vi "GT Get Prf Vel.vi"(6 "pClock":u32, 7 "count":i16, 8 "error in (no error)":errorcluster caption="错误输入（无错误）", 10 "profile":i16, 11 "cardNum":i16) -> (0 "error out":errorcluster caption="错误输出", 1 "pValue out":dbl[](array[numeric]), 3 "function return":i16, 4 "pClock out":u32)   [LabVIEW 2014, in "gts.lvlib"]
doc: "GT_API GT_GetPrfVel(short cardNum,short profile,double *pValue,short count=1,unsigned long *pClock=NULL);"
uses:
  gts.lvlib
  gts.dll
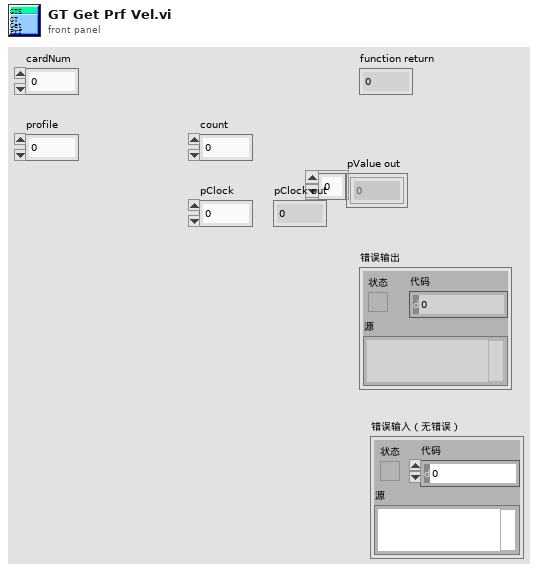
[diagram p1: front panel]
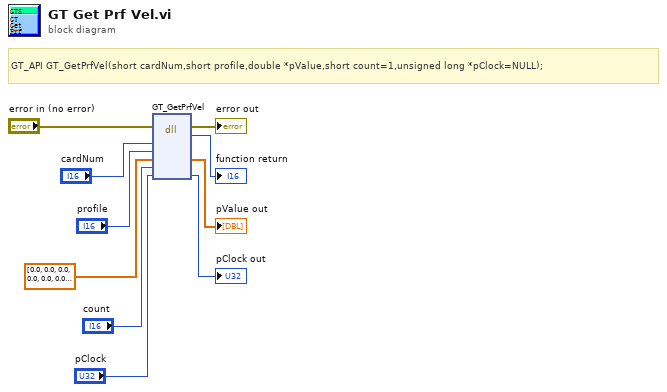
[diagram p0: block diagram]
diagram:
  # "GT_API GT_GetPrfVel(short cardNum,short profile,double *pValue,short count=1,unsigned long *pClock=NULL);"
  n1 = dll-call lib="PTH2?abs D\t王淼清$控制卡常用功能例程(Labview)gts.*" fn="GT_GetPrfVel"(error in="error in (no error)", "cardNum"="cardNum", "profile"="profile", "pValue"=dbl[] [0.0, 0.0, 0.0, 0.0, 0.0, 0.0, 0.0, 1.0], "count"="count", "pClock"="pClock") -> (error out=→"error out":errorcluster, "返回类型"=→"function return":i16, "pValue"=→"pValue out":dbl[], "pClock"=→"pClock out":u32)  [unwired: 5 in, 1 out]
